vi "Parse MSG.vi"(8 "error in":errorcluster, 10 "message type":T2, 11 "stripped message":string) -> (0 "error out":errorcluster, 2 "bytes to read":i32, 3 "header length":i32, 5 "nats message":T1)   [LabVIEW 2013, in "NATS Core.lvlib"]
doc: "Parses the individual properties specified in the MSG string, not including the as-yet unread payload."
uses:
  NATS Core.lvlib
  Controls/msg type.ctl
  Controls/nats message.ctl
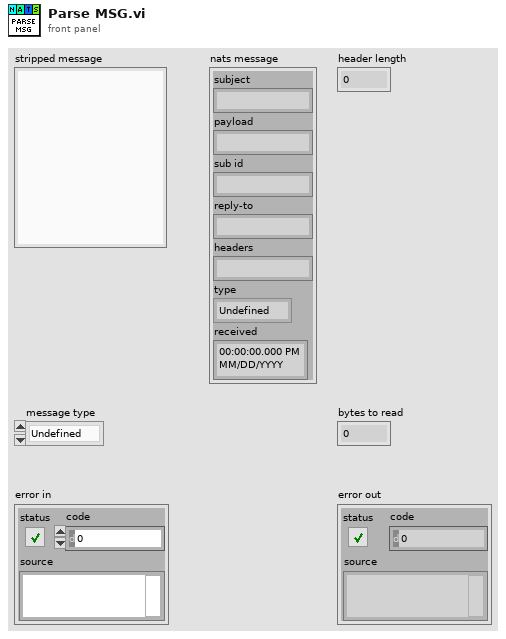
[diagram p1: front panel]
types:
  T1 = typedef "NATS Core.lvlib/nats message.ctl" = cluster{"subject":string, "payload":string, "sub id":string, "reply-to":string, "headers":string, "type":T2, "received":timestamp}
  T2 = typedef "NATS Core.lvlib/msg type.ctl" = enum16{"Undefined", "MSG", "HMSG", "+OK", "PING", "PONG", "-ERR", "INFO"}
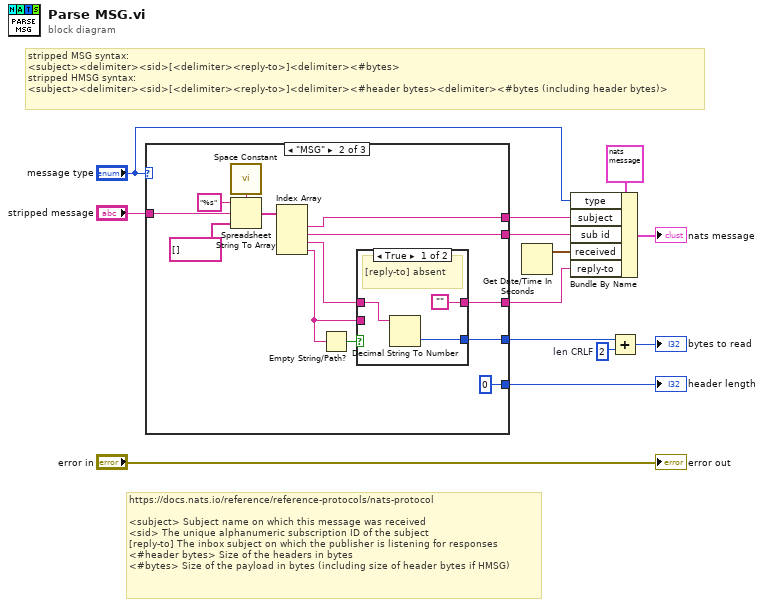
[diagram p0: block diagram]
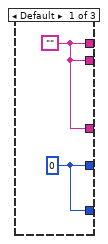
[diagram p2: hidden frame]
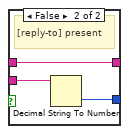
[diagram p3: hidden frame]
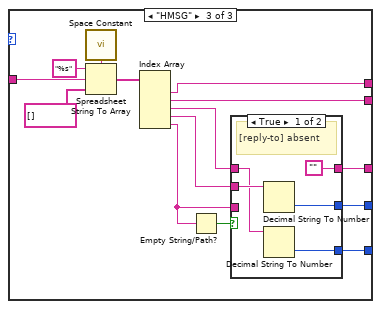
[diagram p4: hidden frame]
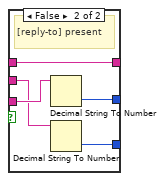
[diagram p5: hidden frame]
diagram:
  w10 = 2  # len CRLF
  # "https://docs.nats.io/reference/reference-protocols/nats-protocol\n\n<subject> Subject name on which this message was received\n<sid> The unique alphanumeric subscription ID of the subject\n[reply-to] The inbox subject on which the publisher is listening for responses\n<#header bytes> Size of the headers in bytes\n<#bytes> Size of the payload in bytes (including size of header bytes if HMSG)"
  # "stripped MSG syntax:\n<subject><delimiter><sid>[<delimiter><reply-to>]<delimiter><#bytes>\nstripped HMSG syntax:\n<subject><delimiter><sid>[<delimiter><reply-to>]<delimiter><#header bytes><delimiter><#bytes (including header bytes)>"
  n1 = case shown="\"MSG\"" "message type" {
    tunnel: [w15 w28 w48] -> w7
    tunnel: [w15 w27 w47] -> w6
    tunnel: "stripped message" -> [_ w26 w46]
    tunnel: [w15 w21 w38] -> w2
    tunnel: [w14 w20 w39] -> w11
    tunnel: [w14 0 w40] -> w12
    frame Default {
      w14 = 0
      w15 = ""
    }
    frame "MSG" {
      n2 = call <vilib>:"Space Constant.vi"() -> ("String"=w16:string)
      n3 = Spreadsheet String To Array(delimiter (Tab)=w16, format string="%s", spreadsheet string=w26, array type (2D Dbl)=string[] []) -> (array=w25:string[])
      n4 = Index Array(array=w25) -> (element #1=w28:string, element #2=w27:string, element #3=w23:string, element #4=w22:string)  [unwired: 4 in]
      n5 = Empty String/Path?(string/path=w22) -> (empty?=w24:bool)
      n6 = case shown="True" w24 {
        tunnel: [w31 w34] -> w20
        tunnel: ["" w32] -> w21
        tunnel: w23 -> [w29 w32]
        tunnel: w22 -> [_ w33]
        frame True {
          # "[reply-to] absent"
          n7 = Decimal String To Number(string=w29) -> (number=w31:i32)  [unwired: 2 in, 1 out]
        }
        frame False {
          # "[reply-to] present"
          n8 = Decimal String To Number(string=w33) -> (number=w34:i32)  [unwired: 2 in, 1 out]
        }
      }
    }
    frame "HMSG" {
      n9 = call <vilib>:"Space Constant.vi"() -> ("String"=w35:string)
      n10 = Spreadsheet String To Array(delimiter (Tab)=w35, format string="%s", spreadsheet string=w46, array type (2D Dbl)=string[] []) -> (array=w45:string[])
      n11 = Index Array(array=w45) -> (element #1=w48:string, element #2=w47:string, element #3=w41:string, element #4=w42:string, element #5=w43:string)  [unwired: 5 in]
      n12 = Empty String/Path?(string/path=w43) -> (empty?=w44:bool)
      n13 = case shown="True" w44 {
        tunnel: [w53 w58] -> w39
        tunnel: w43 -> [_ w57]
        tunnel: w42 -> [w52 w55]
        tunnel: ["" w56] -> w38
        tunnel: w41 -> [w50 w56]
        tunnel: [w49 w54] -> w40
        frame True {
          # "[reply-to] absent"
          n14 = Decimal String To Number(string=w52) -> (number=w53:i32)  [unwired: 2 in, 1 out]
          n15 = Decimal String To Number(string=w50) -> (number=w49:i32)  [unwired: 2 in, 1 out]
        }
        frame False {
          # "[reply-to] present"
          n16 = Decimal String To Number(string=w57) -> (number=w58:i32)  [unwired: 2 in, 1 out]
          n17 = Decimal String To Number(string=w55) -> (number=w54:i32)  [unwired: 2 in, 1 out]
        }
      }
    }
  }
  "header length" <- w12
  n18 = Get Date/Time In Seconds() -> (seconds since 1Jan1904=w3:timestamp)
  n19 = Bundle By Name(cluster=T1 {"subject"="", "payload"="", "sub id"="", "reply-to"="", "headers"="", "type"=enum."Undefined", "received"=timestamp(0 s since 1904-01-01)} ("nats message"), "type"="message type", "subject"=w7, "sub id"=w6, "received"=w3, "reply-to"=w2) -> (→"nats message":T1)
  n20 = Add(x=w11, y=w10) -> (x+y=→"bytes to read":i32)
  "error out" <- "error in"
